vi "trame_ana_save.vi"(11 "Chaîne":string) -> (3 "Instruction":string)   [LabVIEW 2020]
doc: "Analyse la trame pour voir dans quel cas on bacsule"
uses:
  <vilib>/regexp/Match Regular Expression.xnode
panel:
  in  "data in":string="data in"
  in  "expression régulière":string="HIOKI,ST5520,[0-9 A-Z , .]*\\$R"
  in  "cmd":string="HIOKI,ST5520,[0-9 A-Z , .]*\\$R"
  in  "flux in":string
  out "flux out":string
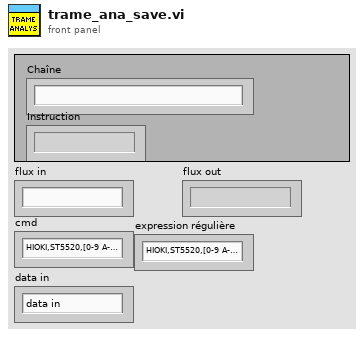
[diagram p1: front panel]
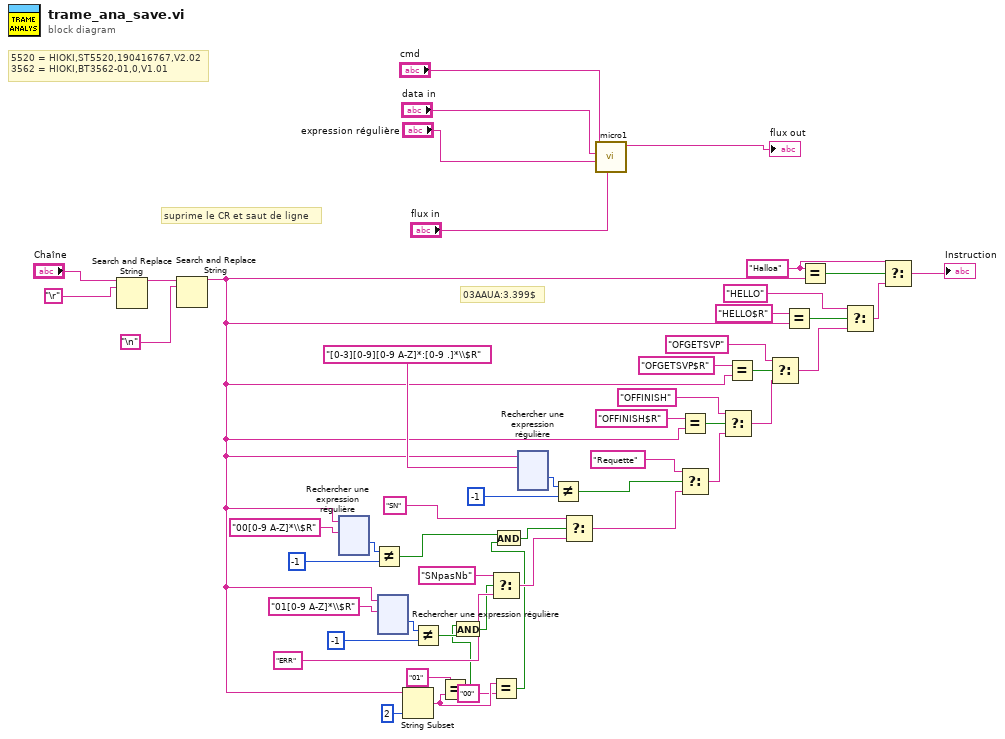
[diagram p0: block diagram]
diagram:
  w29 = "Halloa" ("x")
  # "5520 = HIOKI,ST5520,190416767,V2.02\n3562 = HIOKI,BT3562-01,0,V1.01"
  # "suprime le CR et saut de ligne"
  # "03AAUA:3.399$"
  n1 = Search and Replace String(input string="Chaîne", search string="\r") -> (result string=w10:string)  [unwired: 6 in, 3 out]
  n2 = Search and Replace String(input string=w10, search string="\n") -> (result string=w6:string)  [unwired: 6 in, 3 out]
  n3 = xnode "Rechercher une expression régulière"("chaîne en entrée"=w6, "expression régulière"="00[0-9 A-Z]*\\$R") -> ("offset après correspondance"=w48:i32)  [unwired: 4 in, 4 out]
  n4 = Not Equal? ("Différents ?")(x=w48, y=-1) -> (x != y?=w14:bool)
  n5 = xnode "Rechercher une expression régulière"("chaîne en entrée"=w6, "expression régulière"="01[0-9 A-Z]*\\$R") -> ("offset après correspondance"=w21:i32)  [unwired: 4 in, 4 out]
  n6 = String Subset ("Sous-ensemble d'une chaîne")(string=w6, length (rest)=2 ("longueur (reste)")) -> (substring=w13:string)  [unwired: 1 in]
  n7 = Not Equal? ("Différents ?")(x=w21, y=-1) -> (x != y?=w20:bool)
  n8 = Equal? ("Égaux ?")(x="01", y=w13) -> (x = y?=w17:bool)
  n9 = And(x=w17, y=w20) -> (x .and. y?=w16:bool)
  n10 = Select ("Sélectionner")(t="SNpasNb" ("cas vrai"), s=w16, f="ERR" ("cas faux")) -> (s? t:f=w25:string)
  n11 = Equal? ("Égaux ?")(x=w13, y="00") -> (x = y?=w11:bool)
  n12 = And(x=w14, y=w11) -> (x .and. y?=w15:bool)
  n13 = xnode "Rechercher une expression régulière"("chaîne en entrée"=w6, "expression régulière"="[0-3][0-9][0-9 A-Z]*:[0-9 .]*\\$R") -> ("offset après correspondance"=w43:i32)  [unwired: 4 in, 4 out]
  n14 = Not Equal? ("Différents ?")(x=w43, y=-1) -> (x != y?=w45:bool)
  n15 = Select ("Sélectionner")(t="SN", s=w15, f=w25) -> (s? t:f=w52:string)
  n16 = call "micro1.vi"("flux in en entrée"="flux in", "expression régulière"="expression régulière", "data in"="data in", "cmd"="cmd") -> ("flux in en sortie"=→"flux out":string)  [unwired: 7 in]
  n17 = Equal? ("Égaux ?")(x="OFFINISH$R", y=w6) -> (x = y?=w39:bool)
  n18 = Select ("Sélectionner")(t="Requette", s=w45, f=w52) -> (s? t:f=w47:string)
  n19 = Select ("Sélectionner")(t="OFFINISH", s=w39, f=w47) -> (s? t:f=w41:string)
  n20 = Equal? ("Égaux ?")(x="OFGETSVP$R", y=w6) -> (x = y?=w35:bool)
  n21 = Select(t="OFGETSVP", s=w35, f=w41) -> (s? t:f=w36:string)
  n22 = Equal? ("Égaux ?")(x="HELLO$R", y=w6) -> (x = y?=w32:bool)
  n23 = Equal? ("Égaux ?")(x=w29, y=w6) -> (x = y?=w30:bool)
  n24 = Select(t="HELLO", s=w32, f=w36) -> (s? t:f=w27:string)
  n25 = Select(t=w29, s=w30, f=w27) -> (s? t:f=→"Instruction":string)
